vi "GetTerms3.vi"(0 "XRef":T12, 1 "State In":T9) -> (14 "Terms":T1)   [LabVIEW 2015, in "Async.xnode"]
doc: "This ability VI is used to describe your terminals to LabVIEW. Terms is an array of clusters describing the XNode's terminals.\n ID: A unique string identifying the terminal.\n Name: The name of the terminal visible to the user. Remember to localize it.\n Type: The data type of the terminal (as a Variant). The data put in the variant will be used as the default for the input terminal if it's left unwired.\n Bounds: A rectangle defining the bounds of the terminal relative to the bounds of the XNode. The bounds must be within the bounds of the XNode, and for whiskers to draw properly, they must be flush with at least one side of the XNode.\n Input?: Indicates whether or not this terminals is an input.\n Required?: Indicates whether the user must wire this terminal for the XNode to not be broken. Ignored on outputs.\n Recommended?: Indicates whether the terminal is recommended.\n Hidden?: Indicates whether the terminal is hidden. When a terminal is hidden, it cannot be wired to via user interaction or scripting. However, if it is already wired to when the hidden flag is changed to true, it will remain wired.\n Adaptive?: Indicates that the term should change to match the type of its source if it is wired.\n Direction?: Indicates what direction the wire stub should point. Choose auto to let LV decide based on the terms bounds being on the nodes edge.\n \n The IDs are used by LabVIEW to keep track of your terminals. When you respecify your terminals, LabVIEW can tell whther terminals are new, deleted, or moved by the unique IDs. The order is irrelevant. If you move a terminal, then any wire connected to it will move with it.\n \n If you want to update your terminals, you should return the UpdateTerms reply in one of your ability VIs.\n\nDefault behavior: None.\n\nThis ability does not provide UI and OS messages are not handled."
uses:
  Async.xnode
  <vilib>/XNodeSupport/XNodeXNodeRef.ctl
  State.ctl
  <vilib>/Utility/miscctls.llb/LVRectTypeDef.ctl
  <vilib>/picture/picture.llb/imagedata.ctl
  <vilib>/XNodeSupport/XNodeTerm3Array.ctl
  <vilib>/XNodeSupport/XNodeTerm3.ctl
  <vilib>/XNodeSupport/XNodeString.ctl
  <vilib>/XNodeSupport/XNodeVariant.ctl
  <vilib>/XNodeSupport/XNodeRect32.ctl
  <vilib>/XNodeSupport/XNodeInt.ctl
  <vilib>/XNodeSupport/XNodeBool.ctl
  <vilib>/XNodeSupport/XNodeTermDirection.ctl
  <vilib>/Utility/Data Type/Type Definitions/Data Type.ctl
  <vilib>/XNodeSupport/NI_XNodeSupport.lvlib
  <vilib>/Utility/Data Type/NI_Data Type.lvlib
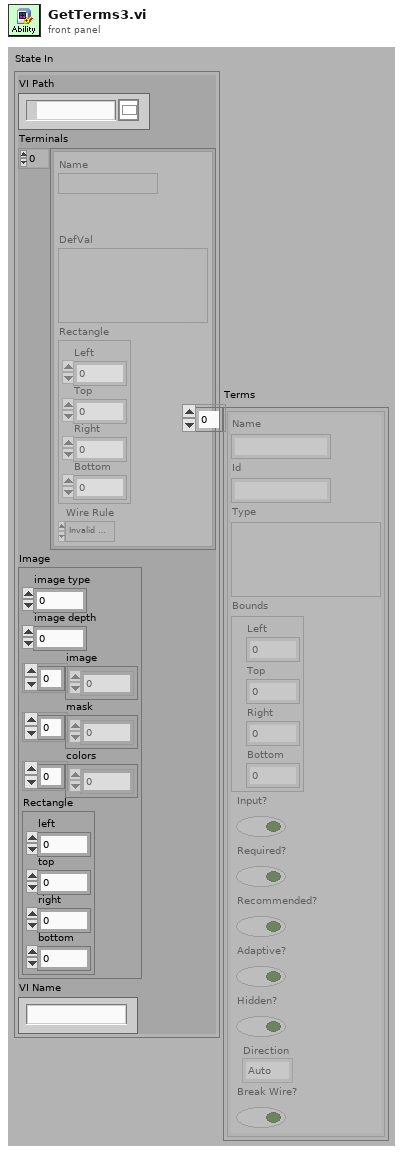
[diagram p1: front panel]
types:
  T1 = typedef "NI_XNodeSupport.lvlib/XNodeTerm3Array.ctl" = T2[]
  T2 = typedef "NI_XNodeSupport.lvlib/XNodeTerm3.ctl" = cluster{"Name":T3, "Id":T3, "Type":T4, "Bounds":T5, "Input?":T7, "Required?":T7, "Recommended?":T7, "Adaptive?":T7, "Hidden?":T7, "Direction":T8, "Break Wire?":T7}
  T3 = typedef "NI_XNodeSupport.lvlib/XNodeString.ctl" = string
  T4 = typedef "NI_XNodeSupport.lvlib/XNodeVariant.ctl" = variant
  T5 = typedef "NI_XNodeSupport.lvlib/XNodeRect32.ctl" = cluster{"Left":T6, "Top":T6, "Right":T6, "Bottom":T6}
  T6 = typedef "NI_XNodeSupport.lvlib/XNodeInt.ctl" = i32
  T7 = typedef "NI_XNodeSupport.lvlib/XNodeBool.ctl" = bool
  T8 = typedef "NI_XNodeSupport.lvlib/XNodeTermDirection.ctl" = enum32{"Auto", "Up", "Down", "Left", "Right", "Center"}
  T9 = typedef "Async.xnode/State.ctl" = cluster{"VI Path":path, "Terminals":cluster{"Name":string, "DefVal":variant, "Rectangle":T10, "Wire Rule":enum16{"Invalid Wire Rule", "Required", "Recommended", "Optional", "Dynamic Dispatch"}}[], "Image":T11, "VI Name":string}
  T10 = typedef "LVRectTypeDef.ctl" = cluster{"Left":i16, "Top":i16, "Right":i16, "Bottom":i16}
  T11 = typedef "imagedata.ctl" = cluster{"image type":i32, "image depth":i32, "image":u8[], "mask":u8[], "colors":u32[], "Rectangle":cluster{"left":i16, "top":i16, "right":i16, "bottom":i16}}
  T12 = typedef "NI_XNodeSupport.lvlib/XNodeXNodeRef.ctl" = refnum<vi>
  T13 = cluster{"Name":string, "DefVal":variant, "Rectangle":T10, "Wire Rule":enum16{"Invalid Wire Rule", "Required", "Recommended", "Optional", "Dynamic Dispatch"}}[]
  T14 = typedef "NI_Data Type.lvlib/Data Type.ctl" = enum8{"Invalid Type", "Void", "I8", "I16", "I32", "I64", "U8", "U16", "U32", "U64", "Single Float", "Double Float", "Extended Float", "Single Complex", "Double Complex", "Extended Complex", "Enum U8", "Enum U16", "Enum U32", "Enum U64", "Single Float With Unit", "Double Float With Unit", "Extended Float With Unit", "Single Complex with Unit", "Double Complex with Unit", "Extended Complex with Unit", "Boolean", "String", "Path", "Picture", "Tag", "Array", "Cluster", "Variant", "LV Variant", "Waveform", "Timestamp", "Digital Waveform", "Digital Data", "ExpressData", "Refnum", "External Data", "VI", "Poly VI", "LabVIEW Class Instance", "Fixed Point"}
  T15 = enum16{"Invalid Wire Rule", "Required", "Recommended", "Optional", "Dynamic Dispatch"}
  T16 = cluster{"Left":bool, "Top":bool, "Right":bool, "Bottom":bool}
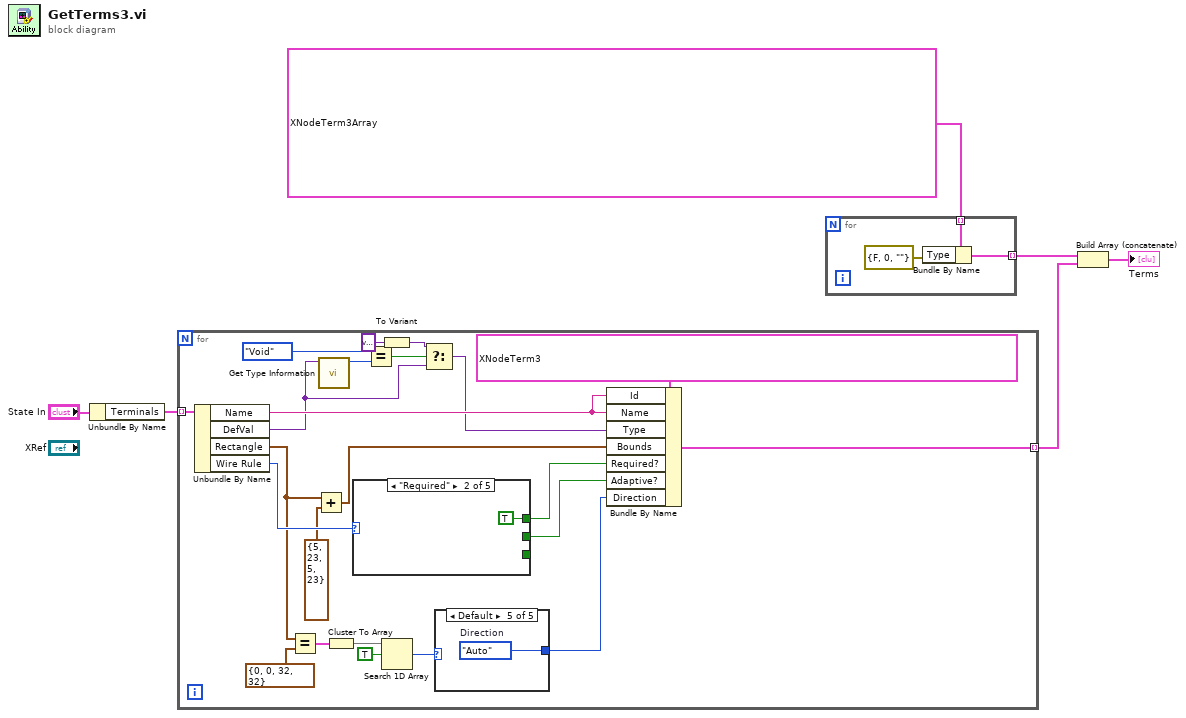
[diagram p0: block diagram]
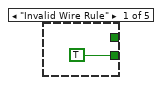
[diagram p2: hidden frame]
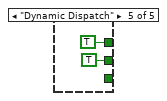
[diagram p5: hidden frame]
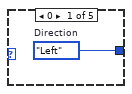
[diagram p6: hidden frame]
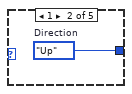
[diagram p7: hidden frame]
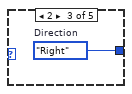
[diagram p8: hidden frame]
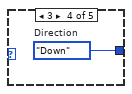
[diagram p9: hidden frame]
diagram:
  n1 = Unbundle By Name("State In") -> ("Terminals"=w5:T13)
  n2 = for {
    tunnel: w5 -> [w29] mode=indexing
    tunnel: [w23] -> w2 mode=indexing
    n3 = Unbundle By Name(w29) -> ("Name"=w21:string, "DefVal"=w14:variant, "Rectangle"=w10:T10, "Wire Rule"=w25:T15)
    n4 = Equal?(x=w10, y=T10 {"Left"=0, "Top"=0, "Right"=32, "Bottom"=32}) -> (x = y?=w11:T16)
    n5 = Add(x=w10, y=T10 {"Left"=5, "Top"=23, "Right"=5, "Bottom"=23}) -> (x+y=w20:T10)
    n6 = call <vilib>:"Get Type Information.vi"("Variant"=w14) -> ("Type"=w18:T14)  [unwired: 6 in, 4 out]
    n7 = Cluster To Array(cluster=w11) -> (array=w28:bool[])
    n8 = case shown="\"Required\"" w25 {
      tunnel: [_ TRUE _ _ TRUE] -> w24
      tunnel: [TRUE _ _ _ _] -> _
      tunnel: [_ _ _ _ TRUE] -> w22
      frame "Invalid Wire Rule" {
      }
      frame "Required" {
      }
      frame "Recommended" {
      }
      frame "Optional" {
      }
      frame "Dynamic Dispatch" {
      }
    }
    n9 = Equal?(x=Data_Type."Void", y=w18) -> (x = y?=w16:bool)
    n10 = To Variant(anything=variant) -> (Variant=w15:variant)
    n11 = Search 1D Array(1D array=w28, element=TRUE) -> (index of element=w27:i32)  [unwired: 1 in]
    n12 = Select(t=w15, s=w16, f=w14) -> (s? t:f=w13:variant)
    n13 = case shown="Default" w27 {
      tunnel: [w34 w35 w36 w37 w38] -> w7
      frame 0 {
        w34 = XNodeTermDirection."Left"  # Direction
      }
      frame 1 {
        w35 = XNodeTermDirection."Up"  # Direction
      }
      frame 2 {
        w36 = XNodeTermDirection."Right"  # Direction
      }
      frame 3 {
        w37 = XNodeTermDirection."Down"  # Direction
      }
      frame Default {
        w38 = XNodeTermDirection."Auto"  # Direction
      }
    }
    n14 = Bundle By Name(cluster=T2 {"Name"="", "Id"="", "Type"=variant, "Bounds"={"Left"=0, "Top"=0, "Right"=0, "Bottom"=0}, "Input?"=TRUE, "Required?"=FALSE, "Recommended?"=FALSE, "Adaptive?"=FALSE, "Hidden?"=FALSE, "Direction"=enum."Auto", "Break Wire?"=FALSE} ("Term 3"), "Id"=w21, "Name"=w21, "Type"=w13, "Bounds"=w20, "Required?"=w24, "Adaptive?"=w22, "Direction"=w7) -> (w23:T2)
  }
  n15 = for {
    tunnel: T1 [{"Name"="Error In", "Id"="ein", "Type"=variant, "Bounds"={"Left"=0, "Top"=9, "Right"=8, "Bottom"=17}, "Input?"=TRUE, "Required?"=FALSE, "Recommended?"=FALSE, "Adaptive?"=FALSE, "Hidden?"=FALSE, "Direction"=enum."Auto", "Break Wire?"=FALSE}, {"Name"="Error Out", "Id"="eout", "Type"=variant, "Bounds"={"Left"=34, "Top"=9, "Right"=42, "Bottom"=17}, "Input?"=FALSE, "Required?"=FALSE, "Recommended?"=FALSE, "Adaptive?"=FALSE, "Hidden?"=FALSE, "Direction"=enum."Auto", "Break Wire?"=FALSE}, {"Name"="VI Ref", "Id"="viref", "Type"=variant, "Bounds"={"Left"=34, "Top"=1, "Right"=42, "Bottom"=8}, "Input?"=FALSE, "Required?"=FALSE, "Recommended?"=FALSE, "Adaptive?"=TRUE, "Hidden?"=FALSE, "Direction"=enum."Right", "Break Wire?"=FALSE}] ("Terms") -> [w41] mode=indexing
    tunnel: [w39] -> w3 mode=indexing
    n16 = Bundle By Name(cluster=w41, "Type"=errorcluster {"status"=FALSE, "code"=0, "source"=""} ("error constant")) -> (w39:T2)
  }
  n17 = Build Array (concatenate)(w3, w2) -> (→"Terms":T2[])
